vi "led显示更新字符串山推.vi"(10 "显示字符":string="山推平地机实验台", 11 "立显/保存":bool=TRUE) -> (3 "发送数据":string)   [LabVIEW 2016]
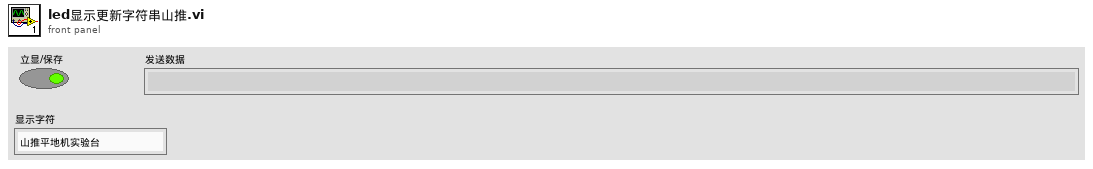
[diagram p1: front panel]
types:
  T1 = enum16{"big-endian, network order", "native, host order", "little-endian"}
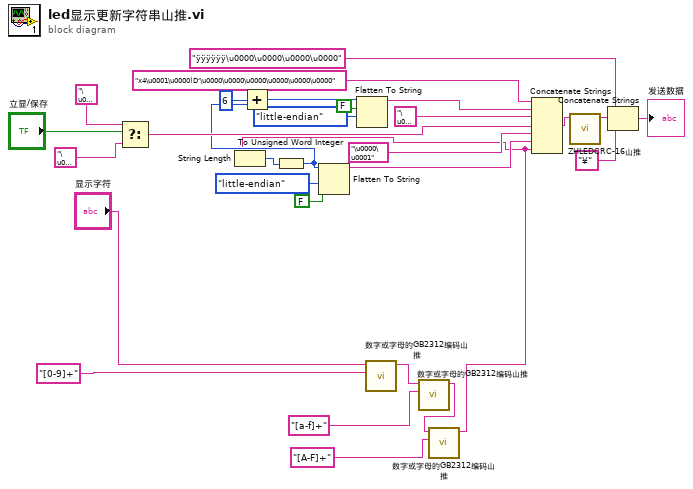
[diagram p0: block diagram]
diagram:
  n1 = Select(t="\u0000" ("关闭AD采样"), s="立显/保存", f="\u0002" ("关闭AD采样")) -> (s? t:f=w29:string)
  n2 = call "数字或字母的GB2312编码山推.vi"("正则表达式"="[0-9]+", "显示字符输入"="显示字符") -> ("显示字符输出"=w2:string)  [unwired: 9 in]
  n3 = call "数字或字母的GB2312编码山推.vi"("正则表达式"="[a-f]+", "显示字符输入"=w2) -> ("显示字符输出"=w4:string)  [unwired: 9 in]
  n4 = call "数字或字母的GB2312编码山推.vi"("正则表达式"="[A-F]+", "显示字符输入"=w4) -> ("显示字符输出"=w1:string)  [unwired: 9 in]
  n5 = String Length(string=w1) -> (length=w12:i32)
  n6 = To Unsigned Word Integer(number=w12) -> (unsigned 16bit integer=w17:u16)
  n7 = Add(x=u16 6, y=w17) -> (x+y=w19:u16)
  n8 = Flatten To String(anything=w17, prepend array or string size? (T)=FALSE ("预置数组或字符串大小？ (T)"), byte order (0:big-endian, network order)=T1."little-endian" ("字节顺序(0:big-endian, network order)")) -> (data string=w14:string)  [unwired: 1 in, 2 out]
  n9 = Flatten To String(anything=w19, prepend array or string size? (T)=FALSE ("预置数组或字符串大小？ (T)"), byte order (0:big-endian, network order)=T1."little-endian" ("字节顺序(0:big-endian, network order)")) -> (data string=w20:string)  [unwired: 1 in, 2 out]
  n10 = Concatenate Strings("x4\u0001\u0000)D‘\u0000\u0000\u0000\u0000\u0000\u0000" ("关闭AD采样"), w20, "\u0001" ("关闭AD采样"), w29, "\u0000\u0001" ("关闭AD采样"), w14, w1) -> (w21:string)
  n11 = call "ZHLEDCRC-16山推.vi"("String"=w21) -> ("String & CRC-16"=w23:string)  [unwired: 8 in, 2 out]
  n12 = Concatenate Strings("ÿÿÿÿÿÿ\u0000\u0000\u0000\u0000" ("关闭AD采样"), w23, "¥" ("关闭AD采样")) -> (→"发送数据":string)
